vi "TDT-Get Hot Block.vi"(0 "Data":T1={"TTankX"=refnum, "TDevAccX"=refnum, "LastTime"=0.0, "error"={"status"=FALSE, "code"=0, "source"=""}, "Block Name"="", "Circuit Tag"="", "Tank Name"="", "NumTicks"=0, "LastTick"=0.0, "Idle?"=FALSE, "Wait (ms)"=1000, "LastArtf"=0.0, "LastTosc"=0.0}, 11 "error in (no error)":errorcluster) -> (8 "HotBlock":string, 10 "TankName":string, 15 "error out":errorcluster)   [LabVIEW 2015]
uses:
  TDT Interface Data.ctl
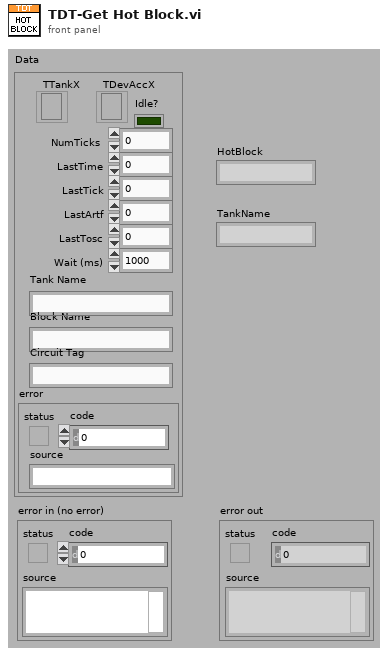
[diagram p1: front panel]
types:
  T1 = typedef "TDT Interface Data.ctl" = cluster{"TTankX":refnum<k7>, "TDevAccX":refnum<k7>, "LastTime":dbl, "error":errorcluster, "Block Name":string, "Circuit Tag":string, "Tank Name":string, "NumTicks":i32, "LastTick":dbl, "Idle?":bool, "Wait (ms)":u32, "LastArtf":dbl, "LastTosc":dbl}
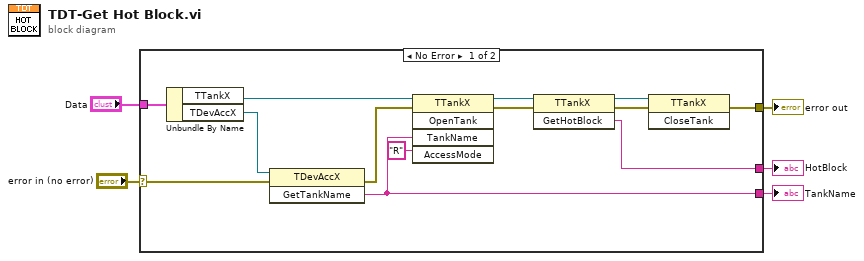
[diagram p0: block diagram]
diagram:
  n1 = case shown="No Error" "error in (no error)" {
    selector: "error in (no error)" -> [w17 w19]
    tunnel: [w18 w19] -> w4
    tunnel: "Data" -> [w14 _]
    tunnel: [w13 _] -> w2
    tunnel: [w6 _] -> w1
    frame No Error {
      n2 = Unbundle By Name(w14) -> ("TTankX"=w15:refnum<k7>, "TDevAccX"=w16:refnum<k7>)
      n3 = invoke class="TDevAccX" method="GetTankName"(reference=w16, error in=w17) -> (error out=w11:errorcluster, "GetTankName"=w6:string)  [unwired: 1 in, 1 out]
      n4 = invoke class="TTankX" method="OpenTank"(reference=w15, error in=w11, "TankName"=w6, "AccessMode"="R") -> (reference out=w12:refnum<k7>, error out=w9:errorcluster)  [unwired: 1 in, 3 out]
      n5 = invoke class="TTankX" method="GetHotBlock"(reference=w12, error in=w9) -> (reference out=w8:refnum<k7>, error out=w7:errorcluster, "GetHotBlock"=w13:string)  [unwired: 1 in]
      n6 = invoke class="TTankX" method="CloseTank"(reference=w8, error in=w7) -> (error out=w18:errorcluster)  [unwired: 1 in, 2 out]
    }
    frame Error {
    }
  }
  "error out" <- w4
  "HotBlock" <- w2
  "TankName" <- w1
